vi "Export header file.vi"(8 "error in (no error)":errorcluster, 11 "CCD in":refnum<class "CCD.lvclass">) -> (0 "error out":errorcluster, 3 "CCD out":refnum<class "CCD.lvclass">)   [LabVIEW 2018, in "CCD.lvclass"]
uses:
  CCD.lvclass
  CCD.lvclass/CCD.ctl
panel:
  out "Camera Setup":T1={"FILENAME"="CH1_009.fits", "OBSERVER"="Anonymous", "PROGrID"="2018A-001", "OBJECT"="UNDEFINED", "NIGHTDIR"="C:\\Users\\observer\\Desktop\\SPARC4 Acquisition Control\\Imagens\\", "CHANNEL"="1", "INSTRUME"="SPARC4", "NEXPSEQ"="1", "SEQINDEX"="1", "OBSTYPE"="UNDEFINED", "READMOD"="UNDEFINED", "READMODE"="Image", "ACQMODE"="Kinetic", "PREAMP"="Gain 1", "READOUT"="30 MHz", "VSHIFT"="4.33", "TRIGGER"="Internal", "EMMODE"="Electron Multiplying", "EMGAIN"="2", "VBIN"="1", "HBIN"="1", "INITLINE"="1", "INITCOL"="1", "FINALLIN"="1024", "FINALCOL"="1024", "KSERLEN"="1", "SHUTTER"="CLOSED", "OPENSHT"="50", "CLOSESHT"="50", "DATE"="2019-03-20T12:18:53.53", "GAIN"="0.0", "GAINERR"="0.0", "RDNOISE"="0.0", "RNOISERR"="0.0", "SKYFIBER"="OFF", "CALFIBER"="OFF", "UTDATE"="2017-10-01T20", "LOCTIME"="2017-10-01T17", "MJD"="0.0", "OBSLON"="0.0", "OBSLAT"="0.0", "OBSALT"="0.0", "EXPTIME"="0", "TELRA"="00:00:00.000", "TELDEC"="+00:00:00.000", "RA"="00:00:00.000", "DEC"="+00:00:00.000", "RA_DEG"="0.0", "DEC_DEG"="0.0", "EPOCH"="2000.00", "HA"="+01:13:05.980.0", "HAD"="0.0", "AIRMASS"="0.0", "AMSTART"="0.0", "AMEND"="0.0", "XOFFSET"="0.000000", "YOFFSET"="0.000000", "PA"="0.0", "CAMFOC"="0.0", "TELFOC"="0.0", "TCSUT"="00:00:00.0", "TCSST"="00:00:00.0", "MOONDIST"="0.0", "MOONALT"="0.0", "MOONPHAS"="0.0", "ADC"="OFF", "ADCSPEED"="0", "CALMIR"="OUT", "GUIDING"="OFF", "GUIDTEXP"="0", "GUIDFREQ"="0", "GUIDOBJX"="0.0", "GUIDOBJY"="0.0", "AVGYCORR"="0.0", "AVGXCORR"="0.0", "GFOCUS"="0.0", "THARLAMP"="OFF", "HALLAMP"="OFF", "AGITATOR"="OFF", "THARMIR"="UNDEFINED", "DSTATUS"="CLOSED", "DPOS"="0.00000", "DTEMP"="0.0", "DHUM"="0.0", "DLAMP"="OFF", "DFLAT"="OFF", "TEMPEXT"="0.0", "PRESSURE"="0.0", "HUMIDITY"="0.0", "WINDDIR"="0.0", "WINDSPEED"="0.0", "SHTTTL"="TTL LOW"}
  out "Camera Setup 2":T2={"FILENAME"="img_000.fits", "NIGHTDIR"="C:\\Users\\observer\\Desktop\\Imagens_CCD\\EXP1\\", "NEXPSEQ"="1", "SEQINDEX"="1", "READMODE"="Image", "ACQMODE"="Kinetic", "PREAMP"="Gain 1", "READOUT"="1 MHz", "VSHIFT"="0.6", "TRIGGER"="Internal", "EMMODE"="Conventional", "EMGAIN"="2", "VBIN"="1", "HBIN"="1", "INITLINE"="1", "INITCOL"="1", "FINALLIN"="1024", "FINALCOL"="1024", "KSERLEN"="1", "SHUTTER"="CLOSED", "OPENSHT"="50", "CLOSESHT"="50", "DATE"="2020-03-26T15:09:07.83", "EXPTIME"="0,000010", "SHTTTL"="TTL LOW", "TEMP"="20", "TEMPST"=""}
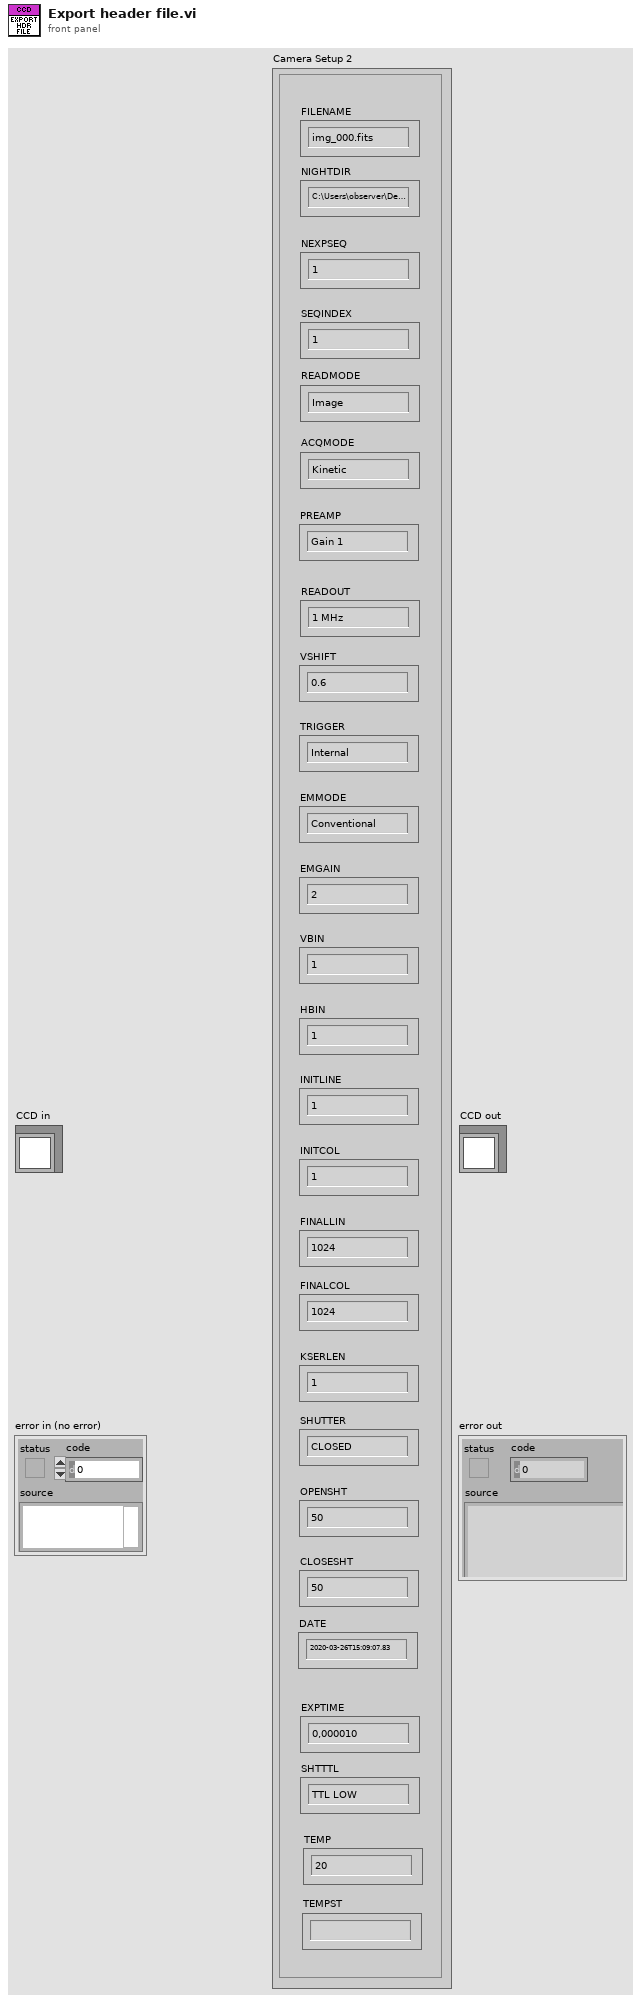
[diagram p1: front panel]
types:
  T1 = cluster{"FILENAME":string, "OBSERVER":string, "PROGrID":string, "OBJECT":string, "NIGHTDIR":string, "CHANNEL":string, "INSTRUME":string, "NEXPSEQ":string, "SEQINDEX":string, "OBSTYPE":string, "READMOD":string, "READMODE":string, "ACQMODE":string, "PREAMP":string, "READOUT":string, "VSHIFT":string, "TRIGGER":string, "EMMODE":string, "EMGAIN":string, "VBIN":string, "HBIN":string, "INITLINE":string, "INITCOL":string, "FINALLIN":string, "FINALCOL":string, "KSERLEN":string, "SHUTTER":string, "OPENSHT":string, "CLOSESHT":string, "DATE":string, "GAIN":string, "GAINERR":string, "RDNOISE":string, "RNOISERR":string, "SKYFIBER":string, "CALFIBER":string, "UTDATE":string, "LOCTIME":string, "MJD":string, "OBSLON":string, "OBSLAT":string, "OBSALT":string, "EXPTIME":string, "TELRA":string, "TELDEC":string, "RA":string, "DEC":string, "RA_DEG":string, "DEC_DEG":string, "EPOCH":string, "HA":string, "HAD":string, "AIRMASS":string, "AMSTART":string, "AMEND":string, "XOFFSET":string, "YOFFSET":string, "PA":string, "CAMFOC":string, "TELFOC":string, "TCSUT":string, "TCSST":string, "MOONDIST":string, "MOONALT":string, "MOONPHAS":string, "ADC":string, "ADCSPEED":string, "CALMIR":string, "GUIDING":string, "GUIDTEXP":string, "GUIDFREQ":string, "GUIDOBJX":string, "GUIDOBJY":string, "AVGYCORR":string, "AVGXCORR":string, "GFOCUS":string, "THARLAMP":string, "HALLAMP":string, "AGITATOR":string, "THARMIR":string, "DSTATUS":string, "DPOS":string, "DTEMP":string, "DHUM":string, "DLAMP":string, "DFLAT":string, "TEMPEXT":string, "PRESSURE":string, "HUMIDITY":string, "WINDDIR":string, "WINDSPEED":string, "SHTTTL":string}
  T2 = cluster{"FILENAME":string, "NIGHTDIR":string, "NEXPSEQ":string, "SEQINDEX":string, "READMODE":string, "ACQMODE":string, "PREAMP":string, "READOUT":string, "VSHIFT":string, "TRIGGER":string, "EMMODE":string, "EMGAIN":string, "VBIN":string, "HBIN":string, "INITLINE":string, "INITCOL":string, "FINALLIN":string, "FINALCOL":string, "KSERLEN":string, "SHUTTER":string, "OPENSHT":string, "CLOSESHT":string, "DATE":string, "EXPTIME":string, "SHTTTL":string, "TEMP":string, "TEMPST":string}
  T3 = enum16{"open", "replace", "create", "open or create", "replace or create", "replace or create with confirmation"}
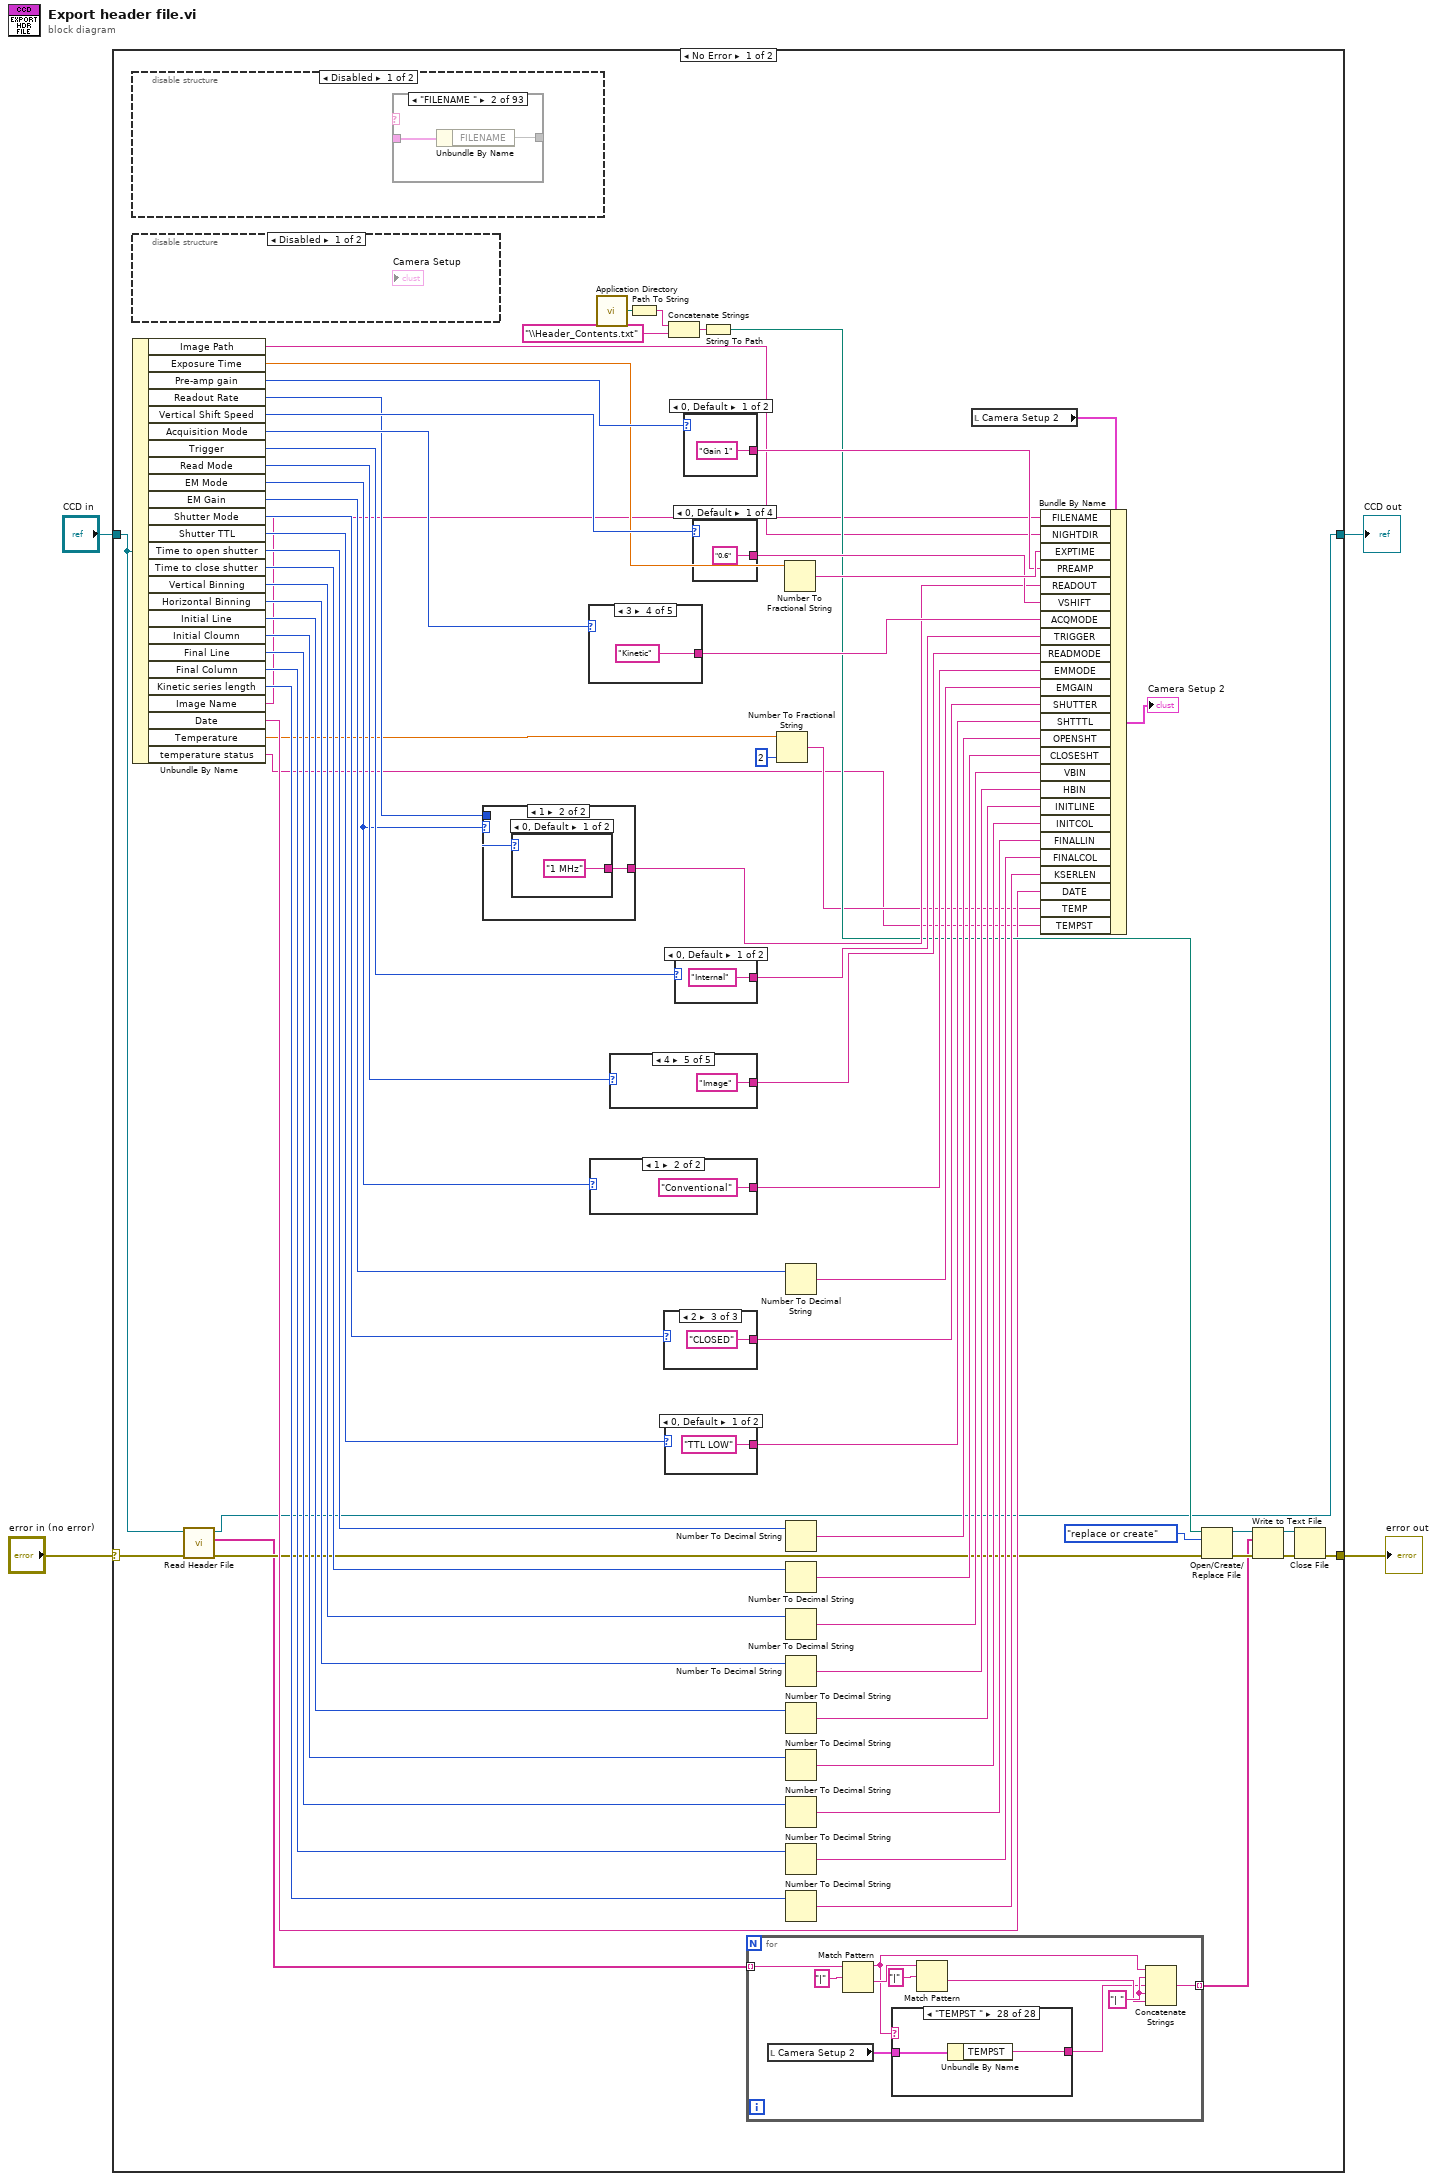
[diagram p0: block diagram]
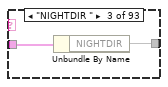
[diagram p4: hidden frame]
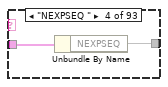
[diagram p5: hidden frame]
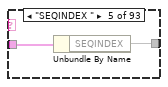
[diagram p6: hidden frame]
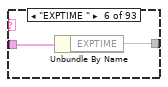
[diagram p7: hidden frame]
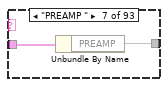
[diagram p8: hidden frame]
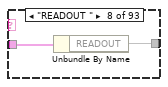
[diagram p9: hidden frame]
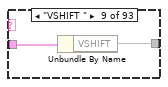
[diagram p10: hidden frame]
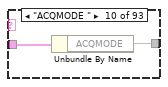
[diagram p11: hidden frame]
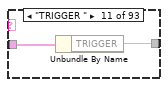
[diagram p12: hidden frame]
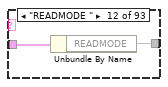
[diagram p13: hidden frame]
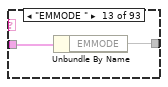
[diagram p14: hidden frame]
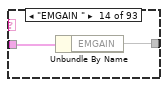
[diagram p15: hidden frame]
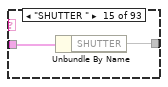
[diagram p16: hidden frame]
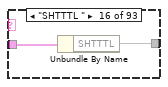
[diagram p17: hidden frame]
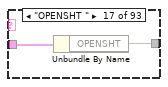
[diagram p18: hidden frame]
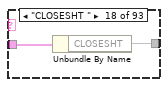
[diagram p19: hidden frame]
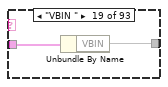
[diagram p20: hidden frame]
diagram:
  n1 = case shown="No Error" "error in (no error)" {
    selector: "error in (no error)" -> [w16 w354]
    tunnel: [w23 w354] -> w2
    tunnel: [w15 w353] -> w1
    tunnel: "CCD in" -> [w17 w353]
    frame No Error {
      n2 = disable-structure shown="Disabled" {
        frame Disabled {
          n3 = case shown="\"FILENAME \"" {
            selector: _ -> [_ _ _ _ _ _ _ _ _ _ _ _ _ _ _ _ _ _ _ _ _ _ _ _ _ _ _ _ _ _ _ _ _ _ _ _ _ _ _ _ _ _ _ _ _ _ _ _ _ _ _ _ _ _ _ _ _ _ _ _ _ _ _ _ _ _ _ _ _ _ _ _ _ _ _ _ _ _ _ _ _ _ _ _ _ _ _ _ _ _ _ _ _]
            tunnel: _ -> [_ w72 w74 w76 w78 w80 w82 w84 w86 w88 w90 w92 w94 w96 w98 w100 w102 w104 w106 w108 w110 w112 w114 w116 w118 w120 w122 w124 w126 w128 w130 w132 w134 w136 w138 w140 w142 w144 w146 w148 w150 w152 w154 w156 w158 w160 w162 w164 w166 w168 w170 w172 w174 w176 w178 w180 w182 w184 w186 w188 w190 w192 w194 w196 w198 w200 w202 w204 w206 w208 w210 w212 w214 w216 w218 w220 w222 w224 w226 w228 w230 w232 w234 w236 w238 w240 w242 w244 w246 w248 w250 w252 w254]
            tunnel: [_ w71 w73 w75 w77 w79 w81 w83 w85 w87 w89 w91 w93 w95 w97 w99 w101 w103 w105 w107 w109 w111 w113 w115 w117 w119 w121 w123 w125 w127 w129 w131 w133 w135 w137 w139 w141 w143 w145 w147 w149 w151 w153 w155 w157 w159 w161 w163 w165 w167 w169 w171 w173 w175 w177 w179 w181 w183 w185 w187 w189 w191 w193 w195 w197 w199 w201 w203 w205 w207 w209 w211 w213 w215 w217 w219 w221 w223 w225 w227 w229 w231 w233 w235 w237 w239 w241 w243 w245 w247 w249 w251 w253] -> _
            frame "False", Default {
            }
            frame "FILENAME " {
              n4 = Unbundle By Name(w72) -> ("FILENAME"=w71)
            }
            frame "NIGHTDIR " {
              n5 = Unbundle By Name(w74) -> ("NIGHTDIR"=w73)
            }
            frame "NEXPSEQ " {
              n6 = Unbundle By Name(w76) -> ("NEXPSEQ"=w75)
            }
            frame "SEQINDEX " {
              n7 = Unbundle By Name(w78) -> ("SEQINDEX"=w77)
            }
            frame "EXPTIME " {
              n8 = Unbundle By Name(w80) -> ("EXPTIME"=w79)
            }
            frame "PREAMP " {
              n9 = Unbundle By Name(w82) -> ("PREAMP"=w81)
            }
            frame "READOUT " {
              n10 = Unbundle By Name(w84) -> ("READOUT"=w83)
            }
            frame "VSHIFT " {
              n11 = Unbundle By Name(w86) -> ("VSHIFT"=w85)
            }
            frame "ACQMODE " {
              n12 = Unbundle By Name(w88) -> ("ACQMODE"=w87)
            }
            frame "TRIGGER " {
              n13 = Unbundle By Name(w90) -> ("TRIGGER"=w89)
            }
            frame "READMODE " {
              n14 = Unbundle By Name(w92) -> ("READMODE"=w91)
            }
            frame "EMMODE " {
              n15 = Unbundle By Name(w94) -> ("EMMODE"=w93)
            }
            frame "EMGAIN " {
              n16 = Unbundle By Name(w96) -> ("EMGAIN"=w95)
            }
            frame "SHUTTER " {
              n17 = Unbundle By Name(w98) -> ("SHUTTER"=w97)
            }
            frame "SHTTTL " {
              n18 = Unbundle By Name(w100) -> ("SHTTTL"=w99)
            }
            frame "OPENSHT " {
              n19 = Unbundle By Name(w102) -> ("OPENSHT"=w101)
            }
            frame "CLOSESHT " {
              n20 = Unbundle By Name(w104) -> ("CLOSESHT"=w103)
            }
            frame "VBIN " {
              n21 = Unbundle By Name(w106) -> ("VBIN"=w105)
            }
            frame "HBIN " {
              n22 = Unbundle By Name(w108) -> ("HBIN"=w107)
            }
            frame "INITLIN " {
              n23 = Unbundle By Name(w110) -> ("INITLINE"=w109)
            }
            frame "INITCOL " {
              n24 = Unbundle By Name(w112) -> ("INITCOL"=w111)
            }
            frame "FINALLIN " {
              n25 = Unbundle By Name(w114) -> ("FINALLIN"=w113)
            }
            frame "FINALCOL " {
              n26 = Unbundle By Name(w116) -> ("FINALCOL"=w115)
            }
            frame "KSERLEN " {
              n27 = Unbundle By Name(w118) -> ("KSERLEN"=w117)
            }
            frame "DATE " {
              n28 = Unbundle By Name(w120) -> ("DATE"=w119)
            }
            frame "INSTRUME " {
              n29 = Unbundle By Name(w122) -> ("INSTRUME"=w121)
            }
            frame "OBSERVER " {
              n30 = Unbundle By Name(w124) -> ("OBSERVER"=w123)
            }
            frame "PROGRID " {
              n31 = Unbundle By Name(w126) -> ("PROGrID"=w125)
            }
            frame "OBJECT " {
              n32 = Unbundle By Name(w128) -> ("OBJECT"=w127)
            }
            frame "CHANNEL " {
              n33 = Unbundle By Name(w130) -> ("CHANNEL"=w129)
            }
            frame "OBSTYPE " {
              n34 = Unbundle By Name(w132) -> ("OBSTYPE"=w131)
            }
            frame "READMOD " {
              n35 = Unbundle By Name(w134) -> ("READMOD"=w133)
            }
            frame "GAIN " {
              n36 = Unbundle By Name(w136) -> ("GAIN"=w135)
            }
            frame "GAINERR " {
              n37 = Unbundle By Name(w138) -> ("GAINERR"=w137)
            }
            frame "RDNOISE " {
              n38 = Unbundle By Name(w140) -> ("RDNOISE"=w139)
            }
            frame "RDNOISERR " {
              n39 = Unbundle By Name(w142) -> ("RNOISERR"=w141)
            }
            frame "SKYFIBER " {
              n40 = Unbundle By Name(w144) -> ("SKYFIBER"=w143)
            }
            frame "CALFIBER " {
              n41 = Unbundle By Name(w146) -> ("CALFIBER"=w145)
            }
            frame "UTDATE " {
              n42 = Unbundle By Name(w148) -> ("UTDATE"=w147)
            }
            frame "LOCTIME " {
              n43 = Unbundle By Name(w150) -> ("LOCTIME"=w149)
            }
            frame "MJD " {
              n44 = Unbundle By Name(w152) -> ("MJD"=w151)
            }
            frame "OBSLON " {
              n45 = Unbundle By Name(w154) -> ("OBSLON"=w153)
            }
            frame "OBSLAT " {
              n46 = Unbundle By Name(w156) -> ("OBSLAT"=w155)
            }
            frame "OBSALT " {
              n47 = Unbundle By Name(w158) -> ("OBSALT"=w157)
            }
            frame "TELRA " {
              n48 = Unbundle By Name(w160) -> ("TELRA"=w159)
            }
            frame "TELDEC " {
              n49 = Unbundle By Name(w162) -> ("TELDEC"=w161)
            }
            frame "RA " {
              n50 = Unbundle By Name(w164) -> ("RA"=w163)
            }
            frame "DEC " {
              n51 = Unbundle By Name(w166) -> ("DEC"=w165)
            }
            frame "RA_DEG " {
              n52 = Unbundle By Name(w168) -> ("RA_DEG"=w167)
            }
            frame "DEC_DEG " {
              n53 = Unbundle By Name(w170) -> ("DEC_DEG"=w169)
            }
            frame "EPOCH " {
              n54 = Unbundle By Name(w172) -> ("EPOCH"=w171)
            }
            frame "HA " {
              n55 = Unbundle By Name(w174) -> ("HA"=w173)
            }
            frame "HAD " {
              n56 = Unbundle By Name(w176) -> ("HAD"=w175)
            }
            frame "AIRMASS " {
              n57 = Unbundle By Name(w178) -> ("AIRMASS"=w177)
            }
            frame "AMSTART " {
              n58 = Unbundle By Name(w180) -> ("AMSTART"=w179)
            }
            frame "AMEND " {
              n59 = Unbundle By Name(w182) -> ("AMEND"=w181)
            }
            frame "XOFFSET " {
              n60 = Unbundle By Name(w184) -> ("XOFFSET"=w183)
            }
            frame "YOFFSET " {
              n61 = Unbundle By Name(w186) -> ("YOFFSET"=w185)
            }
            frame "PA " {
              n62 = Unbundle By Name(w188) -> ("PA"=w187)
            }
            frame "CAMFOC " {
              n63 = Unbundle By Name(w190) -> ("CAMFOC"=w189)
            }
            frame "TELFOC " {
              n64 = Unbundle By Name(w192) -> ("TELFOC"=w191)
            }
            frame "TCSUT " {
              n65 = Unbundle By Name(w194) -> ("TCSUT"=w193)
            }
            frame "TCSST " {
              n66 = Unbundle By Name(w196) -> ("TCSST"=w195)
            }
            frame "MOONDIST " {
              n67 = Unbundle By Name(w198) -> ("MOONDIST"=w197)
            }
            frame "MOONALT " {
              n68 = Unbundle By Name(w200) -> ("MOONALT"=w199)
            }
            frame "MOONPHAS " {
              n69 = Unbundle By Name(w202) -> ("MOONPHAS"=w201)
            }
            frame "ADC " {
              n70 = Unbundle By Name(w204) -> ("ADC"=w203)
            }
            frame "ADCSPEED " {
              n71 = Unbundle By Name(w206) -> ("ADCSPEED"=w205)
            }
            frame "CALMIR " {
              n72 = Unbundle By Name(w208) -> ("CALMIR"=w207)
            }
            frame "GUIDING " {
              n73 = Unbundle By Name(w210) -> ("GUIDING"=w209)
            }
            frame "GUIDTEXP " {
              n74 = Unbundle By Name(w212) -> ("GUIDTEXP"=w211)
            }
            frame "GUIDFREQ " {
              n75 = Unbundle By Name(w214) -> ("GUIDFREQ"=w213)
            }
            frame "GUIDOBJX " {
              n76 = Unbundle By Name(w216) -> ("GUIDOBJX"=w215)
            }
            frame "GUIDOBJY" {
              n77 = Unbundle By Name(w218) -> ("GUIDOBJY"=w217)
            }
            frame "AVGYCORR " {
              n78 = Unbundle By Name(w220) -> ("AVGYCORR"=w219)
            }
            frame "AVGXCORR " {
              n79 = Unbundle By Name(w222) -> ("AVGXCORR"=w221)
            }
            frame "GFOCUS " {
              n80 = Unbundle By Name(w224) -> ("GFOCUS"=w223)
            }
            frame "THARLAMP " {
              n81 = Unbundle By Name(w226) -> ("THARLAMP"=w225)
            }
            frame "HALLAMP " {
              n82 = Unbundle By Name(w228) -> ("HALLAMP"=w227)
            }
            frame "AGITATOR " {
              n83 = Unbundle By Name(w230) -> ("AGITATOR"=w229)
            }
            frame "THARMIR " {
              n84 = Unbundle By Name(w232) -> ("THARMIR"=w231)
            }
            frame "DSTATUS " {
              n85 = Unbundle By Name(w234) -> ("DSTATUS"=w233)
            }
            frame "DPOS " {
              n86 = Unbundle By Name(w236) -> ("DPOS"=w235)
            }
            frame "DTEMP " {
              n87 = Unbundle By Name(w238) -> ("DTEMP"=w237)
            }
            frame "DHUM " {
              n88 = Unbundle By Name(w240) -> ("DHUM"=w239)
            }
            frame "DLAMP " {
              n89 = Unbundle By Name(w242) -> ("DLAMP"=w241)
            }
            frame "DFLAT " {
              n90 = Unbundle By Name(w244) -> ("DFLAT"=w243)
            }
            frame "TEMPEXT " {
              n91 = Unbundle By Name(w246) -> ("TEMPEXT"=w245)
            }
            frame "PRESSURE " {
              n92 = Unbundle By Name(w248) -> ("PRESSURE"=w247)
            }
            frame "HUMIDITY " {
              n93 = Unbundle By Name(w250) -> ("HUMIDITY"=w249)
            }
            frame "WINDIR " {
              n94 = Unbundle By Name(w252) -> ("WINDDIR"=w251)
            }
            frame "WINDSPEED " {
              n95 = Unbundle By Name(w254) -> ("WINDSPEED"=w253)
            }
          }
        }
        frame Enabled {
        }
      }
      n96 = disable-structure shown="Disabled" {
        frame Disabled {
        }
        frame Enabled {
        }
      }
      n97 = Unbundle By Name(w17) -> ("Image Path"=w13:string, "Exposure Time"=w30:dbl, "Pre-amp gain"=w70:u8, "Readout Rate"=w32:u8, "Vertical Shift Speed"=w69:u8, "Acquisition Mode"=w68:u8, "Trigger"=w67:u8, "Read Mode"=w66:u8, "EM Mode"=w33:u8, "EM Gain"=w65:u32, "Shutter Mode"=w64:u8, "Shutter TTL"=w63:u8, "Time to open shutter"=w62:u16, "Time to close shutter"=w61:u16, "Vertical Binning"=w59:u16, "Horizontal Binning"=w60:u16, "Initial Line"=w58:u16, "Initial Cloumn"=w57:u16, "Final Line"=w56:u16, "Final Column"=w55:u16, "Kinetic series length"=w34:u32, "Image Name"=w14:string, "Date"=w20:string, "Temperature"=w10:dbl, "temperature status"=w8:string)
      n98 = call "Read Header File.vi"("error in (no error)"=w16, "CCD in"=w17) -> ("error out"=w19:errorcluster, "Header Contents"=w18:string[], "CCD out"=w15:refnum<class "CCD.lvclass">)  [unwired: 7 in]
      n99 = case shown="1" w33 {
        tunnel: w32 -> [w320 w326]
        tunnel: [w319 w325] -> w31
        frame 0, Default {
          n100 = case shown="2" w320 {
            tunnel: ["30 MHz" ("units") "20 MHz" ("units") "10 MHz" ("units") "1 MHz" ("units")] -> w319
            frame 0, Default {
            }
            frame 1 {
            }
            frame 2 {
            }
            frame 3 {
            }
          }
        }
        frame 1 {
          n101 = case shown="0, Default" w326 {
            tunnel: ["1 MHz" ("units") "0.1 MHz" ("units")] -> w325
            frame 0, Default {
            }
            frame 1 {
            }
          }
        }
      }
      n102 = case shown="3" w68 {
        tunnel: [_ "Single" ("units") "Accumulate" ("units") "Kinetic" ("units") "Fast Kinetic" ("units")] -> w51
        frame 0, Default {
        }
        frame 1 {
        }
        frame 2 {
        }
        frame 3 {
        }
        frame 4 {
        }
      }
      n103 = case shown="1" w33 {
        tunnel: ["Electron Multiplying" ("units") "Conventional" ("units")] -> w48
        frame 0, Default {
        }
        frame 1 {
        }
      }
      n104 = call <vilib>:"Application Directory.vi"() -> ("Application Directory"=w7:path)
      n105 = case shown="4" w66 {
        tunnel: ["Full Vertical Binning" ("units") "Multi-Track" ("units") "Random-Track" ("units") "Single-Track" ("units") "Image" ("units")] -> w49
        frame 0, Default {
        }
        frame 1 {
        }
        frame 2 {
        }
        frame 3 {
        }
        frame 4 {
        }
      }
      n106 = Path To String(path=w7) -> (string=w6:string)
      n107 = case shown="2" w64 {
        tunnel: ["Fully Auto" ("units") "OPEN" ("units") "CLOSED" ("units")] -> w46
        frame 0, Default {
        }
        frame 1 {
        }
        frame 2 {
        }
      }
      n108 = case shown="0, Default" w63 {
        tunnel: ["TTL LOW" ("units") "TTL High" ("units")] -> w45
        frame 0, Default {
        }
        frame 1 {
        }
      }
      n109 = Concatenate Strings(w6, "\\Header_Contents.txt" ("string")) -> (w11:string)
      n110 = case shown="0, Default" w67 {
        tunnel: ["Internal" ("units") "External" ("units")] -> w50
        frame 0, Default {
        }
        frame 1 {
        }
      }
      n111 = case shown="0, Default" w70 {
        tunnel: ["Gain 1" ("units") "Gain 2" ("units")] -> w44
        frame 0, Default {
        }
        frame 1 {
        }
      }
      n112 = case shown="0, Default" w69 {
        tunnel: ["0.6" ("units") "1.13" ("units") "2.2" ("units") "4.33" ("units")] -> w52
        frame 0, Default {
        }
        frame 1 {
        }
        frame 2 {
        }
        frame 3 {
        }
      }
      n113 = String To Path(string=w11) -> (path=w26:path)
      n114 = for {
        tunnel: w18 -> [w264] mode=indexing
        tunnel: [w257] -> w22 mode=indexing
        w261 = "| " ("regular expression")
        n115 = local read "Camera Setup 2"() -> (w259:T2)
        n116 = Match Pattern(string=w264, regular expression="|") -> (before substring=w255:string, after substring=w256:string)  [unwired: 1 in, 2 out]
        n117 = case shown="\"TEMPST \"" w255 {
          tunnel: w259 -> [_ w266 w268 w270 w272 w274 w276 w278 w280 w282 w284 w286 w288 w290 w292 w294 w296 w298 w300 w302 w304 w306 w308 w310 w312 w314 w316 w318]
          tunnel: [_ w265 w267 w269 w271 w273 w275 w277 w279 w281 w283 w285 w287 w289 w291 w293 w295 w297 w299 w301 w303 w305 w307 w309 w311 w313 w315 w317] -> w258
          frame "False", Default {
          }
          frame "FILENAME " {
            n118 = Unbundle By Name(w266) -> ("FILENAME"=w265:string)
          }
          frame "NIGHTDIR " {
            n119 = Unbundle By Name(w268) -> ("NIGHTDIR"=w267:string)
          }
          frame "NEXPSEQ " {
            n120 = Unbundle By Name(w270) -> ("NEXPSEQ"=w269:string)
          }
          frame "SEQINDEX " {
            n121 = Unbundle By Name(w272) -> ("SEQINDEX"=w271:string)
          }
          frame "EXPTIME " {
            n122 = Unbundle By Name(w274) -> ("EXPTIME"=w273:string)
          }
          frame "PREAMP " {
            n123 = Unbundle By Name(w276) -> ("PREAMP"=w275:string)
          }
          frame "READOUT " {
            n124 = Unbundle By Name(w278) -> ("READOUT"=w277:string)
          }
          frame "VSHIFT " {
            n125 = Unbundle By Name(w280) -> ("VSHIFT"=w279:string)
          }
          frame "ACQMODE " {
            n126 = Unbundle By Name(w282) -> ("ACQMODE"=w281:string)
          }
          frame "TRIGGER " {
            n127 = Unbundle By Name(w284) -> ("TRIGGER"=w283:string)
          }
          frame "READMODE " {
            n128 = Unbundle By Name(w286) -> ("READMODE"=w285:string)
          }
          frame "EMMODE " {
            n129 = Unbundle By Name(w288) -> ("EMMODE"=w287:string)
          }
          frame "EMGAIN " {
            n130 = Unbundle By Name(w290) -> ("EMGAIN"=w289:string)
          }
          frame "SHUTTER " {
            n131 = Unbundle By Name(w292) -> ("SHUTTER"=w291:string)
          }
          frame "SHTTTL " {
            n132 = Unbundle By Name(w294) -> ("SHTTTL"=w293:string)
          }
          frame "OPENSHT " {
            n133 = Unbundle By Name(w296) -> ("OPENSHT"=w295:string)
          }
          frame "CLOSESHT " {
            n134 = Unbundle By Name(w298) -> ("CLOSESHT"=w297:string)
          }
          frame "VBIN " {
            n135 = Unbundle By Name(w300) -> ("VBIN"=w299:string)
          }
          frame "HBIN " {
            n136 = Unbundle By Name(w302) -> ("HBIN"=w301:string)
          }
          frame "INITLIN " {
            n137 = Unbundle By Name(w304) -> ("INITLINE"=w303:string)
          }
          frame "INITCOL " {
            n138 = Unbundle By Name(w306) -> ("INITCOL"=w305:string)
          }
          frame "FINALLIN " {
            n139 = Unbundle By Name(w308) -> ("FINALLIN"=w307:string)
          }
          frame "FINALCOL " {
            n140 = Unbundle By Name(w310) -> ("FINALCOL"=w309:string)
          }
          frame "KSERLEN " {
            n141 = Unbundle By Name(w312) -> ("KSERLEN"=w311:string)
          }
          frame "DATE " {
            n142 = Unbundle By Name(w314) -> ("DATE"=w313:string)
          }
          frame "TEMP " {
            n143 = Unbundle By Name(w316) -> ("TEMP"=w315:string)
          }
          frame "TEMPST " {
            n144 = Unbundle By Name(w318) -> ("TEMPST"=w317:string)
          }
        }
        n145 = Match Pattern(string=w256, regular expression="|") -> (after substring=w260:string)  [unwired: 1 in, 3 out]
        n146 = Concatenate Strings(w255, w261, w258, w261, w260) -> (w257:string)
      }
      n147 = Number To Fractional String(number=w10, precision (6)=i16 2) -> (F-format string=w9:string)  [unwired: 2 in]
      n148 = Number To Fractional String(number=w30) -> (F-format string=w53:string)  [unwired: 3 in]
      n149 = Number To Decimal String(number=w65) -> (decimal integer string=w47:string)  [unwired: 1 in]
      n150 = Number To Decimal String(number=w62) -> (decimal integer string=w43:string)  [unwired: 1 in]
      n151 = Number To Decimal String(number=w61) -> (decimal integer string=w42:string)  [unwired: 1 in]
      n152 = Number To Decimal String(number=w59) -> (decimal integer string=w41:string)  [unwired: 1 in]
      n153 = Number To Decimal String(number=w60) -> (decimal integer string=w40:string)  [unwired: 1 in]
      n154 = Number To Decimal String(number=w58) -> (decimal integer string=w39:string)  [unwired: 1 in]
      n155 = Number To Decimal String(number=w57) -> (decimal integer string=w38:string)  [unwired: 1 in]
      n156 = Number To Decimal String(number=w56) -> (decimal integer string=w37:string)  [unwired: 1 in]
      n157 = Number To Decimal String(number=w55) -> (decimal integer string=w36:string)  [unwired: 1 in]
      n158 = Number To Decimal String(number=w34) -> (decimal integer string=w35:string)  [unwired: 1 in]
      n159 = local read "Camera Setup 2"() -> (w54:T2)
      n160 = Bundle By Name(cluster=w54, "FILENAME"=w14, "NIGHTDIR"=w13, "EXPTIME"=w53, "PREAMP"=w44, "READOUT"=w31, "VSHIFT"=w52, "ACQMODE"=w51, "TRIGGER"=w50, "READMODE"=w49, "EMMODE"=w48, "EMGAIN"=w47, "SHUTTER"=w46, "SHTTTL"=w45, "OPENSHT"=w43, "CLOSESHT"=w42, "VBIN"=w41, "HBIN"=w40, "INITLINE"=w39, "INITCOL"=w38, "FINALLIN"=w37, "FINALCOL"=w36, "KSERLEN"=w35, "DATE"=w20, "TEMP"=w9, "TEMPST"=w8) -> (→"Camera Setup 2":T2)
      n161 = Open/Create/Replace File(file path (use dialog)=w26, error in=w19, operation (0:open)=T3."replace or create") -> (refnum out=w27:refnum<file>, error out=w28:errorcluster)  [unwired: 3 in, 1 out]
      n162 = Write to Text File(file (use dialog)=w27, text=w22, error in=w28) -> (refnum out=w24:refnum<file>, error out=w25:errorcluster)  [unwired: 1 in, 1 out]
      n163 = Close File(refnum=w24, error in=w25) -> (error out=w23:errorcluster)  [unwired: 1 out]
    }
    frame Error {
    }
  }
  "error out" <- w2
  "CCD out" <- w1
